vi "scanSpecificationToVolumeSettings.vi"(1 "scan specification":T2={"x amplitude"=100, "x resolution (pixels)"=28, "x offset fly-forward (iterations)"=50, "x offset fly-back (iterations)"=100, "y resolution (nr. of lines)"=80, "y step size"=30, "iterations per pixel"=5, "number of frames"=80, "y offset (pixels)"=0, "number of y-brake lines  (before y-fly-back)"=0, "number y-brake lines (after y-fly-back)"=40, "number of y-fly-back steps"=0, "lines per z step"=1, "number of z/intensity tuples"=228, "number of repetitions (volumes or planes)"=1000, "z step size derived"=32, "choose the beginning of z scan"=FALSE, "number of frames (settings)"=80, "FPGA trajectory?"=TRUE, "Pockels cell voltage (bits)"=0, "Vy min(bits)"=0, "Vz min(bits)"=0}) -> (0 "volume info":T1)   [LabVIEW 2010]
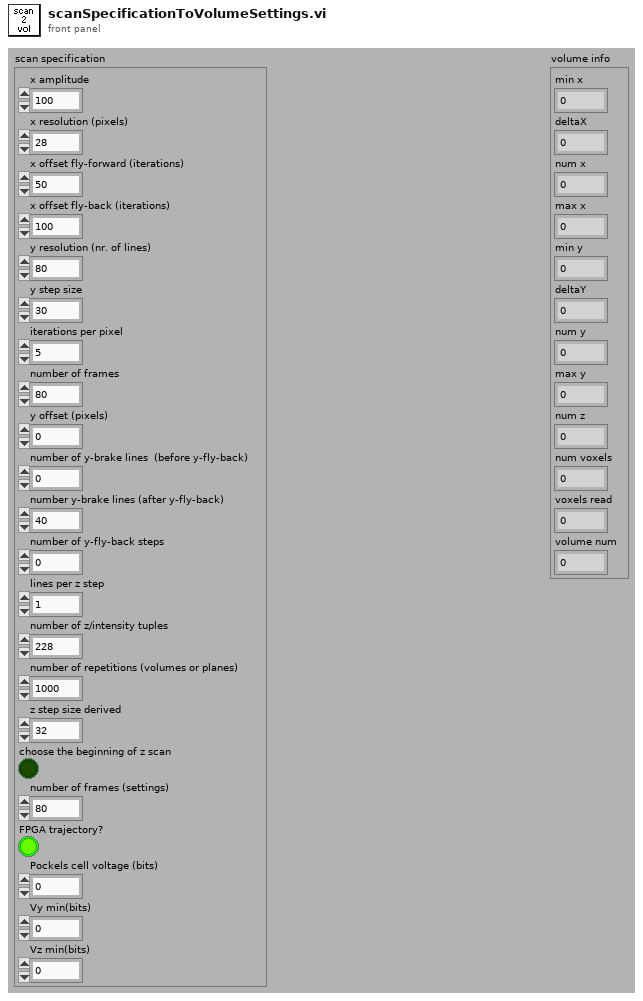
[diagram p1: front panel]
types:
  T1 = cluster{"min x":i16, "deltaX":dbl, "num x":u32, "max x":i16, "min y":i16, "deltaY":dbl, "num y":u32, "max y":i16, "num z":u32, "num voxels":u32, "voxels read":u32, "volume num":u32}
  T2 = cluster{"x amplitude":u16, "x resolution (pixels)":u16, "x offset fly-forward (iterations)":u16, "x offset fly-back (iterations)":u16, "y resolution (nr. of lines)":u16, "y step size":u16, "iterations per pixel":u16, "number of frames":i32, "y offset (pixels)":u16, "number of y-brake lines  (before y-fly-back)":u16, "number y-brake lines (after y-fly-back)":u16, "number of y-fly-back steps":u16, "lines per z step":u16, "number of z/intensity tuples":u16, "number of repetitions (volumes or planes)":i32, "z step size derived":u16, "choose the beginning of z scan":bool, "number of frames (settings)":i32, "FPGA trajectory?":bool, "Pockels cell voltage (bits)":i16, "Vy min(bits)":i16, "Vz min(bits)":i16}
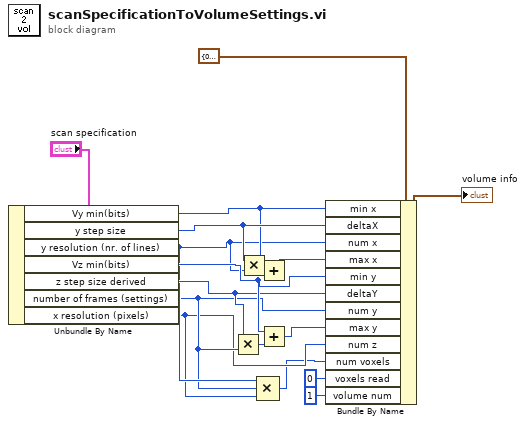
[diagram p0: block diagram]
diagram:
  n1 = Unbundle By Name("scan specification") -> ("Vy min(bits)"=w12:i16, "y step size"=w14:u16, "y resolution (nr. of lines)"=w5:u16, "Vz min(bits)"=w9:i16, "z step size derived"=w6:u16, "number of frames (settings)"=w4:i32, "x resolution (pixels)"=w3:u16)
  n2 = Multiply(x=w6, y=w4) -> (x*y=w10:i32)
  n3 = Multiply(x=w14, y=w5) -> (x*y=w15:u16)
  n4 = Compound Arithmetic op=MULTIPLY(w5, w4, w3) -> (w2:i32)
  n5 = Add(x=w15, y=w12) -> (x+y=w13:u16)
  n6 = Add(x=w9, y=w10) -> (x+y=w11:i32)
  n7 = Bundle By Name(cluster=T1 {"min x"=0, "deltaX"=0.0, "num x"=0, "max x"=0, "min y"=0, "deltaY"=0.0, "num y"=0, "max y"=0, "num z"=0, "num voxels"=0, "voxels read"=0, "volume num"=0} ("element"), "min x"=w12, "deltaX"=w14, "num x"=w5, "max x"=w13, "min y"=w9, "deltaY"=w6, "num y"=w4, "max y"=w11, "num z"=w3, "num voxels"=w2, "voxels read"=u32 0, "volume num"=u32 1) -> (→"volume info":T1)
